vi "Parse Test.vi"() -> ()   [LabVIEW 2015]
uses:
  lib/TOML Value.ctl
  lib/TOML.lvlib
panel:
  out "Parsed Data":T1 {"owner"."dob" format="%<%.3X%z\n%x>T"}
  out "TOML String":string
  in  "Tree":string(tree)
  in  "TOML String":string="# This is a TOML document.\n\ntitle = \"TOML Example\"\n\n[owner]\nname = \"David Taylor\"\ndob = 1991-07-17T07:12:00-07:00 # First class dates\n\n[database]\nserver = \"192.168.1.1\"\nports = [ 8001, 8001, 8002 ]\nconnection_max = 5000\nenabled = true\n\n[servers]\n\n  # Indentation (tabs and/or spaces) is allowed but not required\n  [servers.alpha]\n  ip = \"10.0.0.1\"\n  dc = \"eqdc10\"\n\n  [servers.beta]\n  ip = \"10.0.0.2\"\n  dc = \"eqdc10\"\n\n[clients]\ndata = [ [\"gamma\", \"delta\"], [1, 2] ]\n\n# Line breaks are OK when inside arrays\nhosts = [\n  \"alpha\",\n  \"omega\"\n]\n\n#inline table\ninline_table = {one = 1, two = 2}\n\n[[array_of_tables]]\nmulti-line-string = \"\"\"\nline one\nline two\"\"\"\n\n[[array_of_tables]]\nmulti-line-literal-string = '''\nliteral strings allow special characters \\ unescaped\nline two'''"
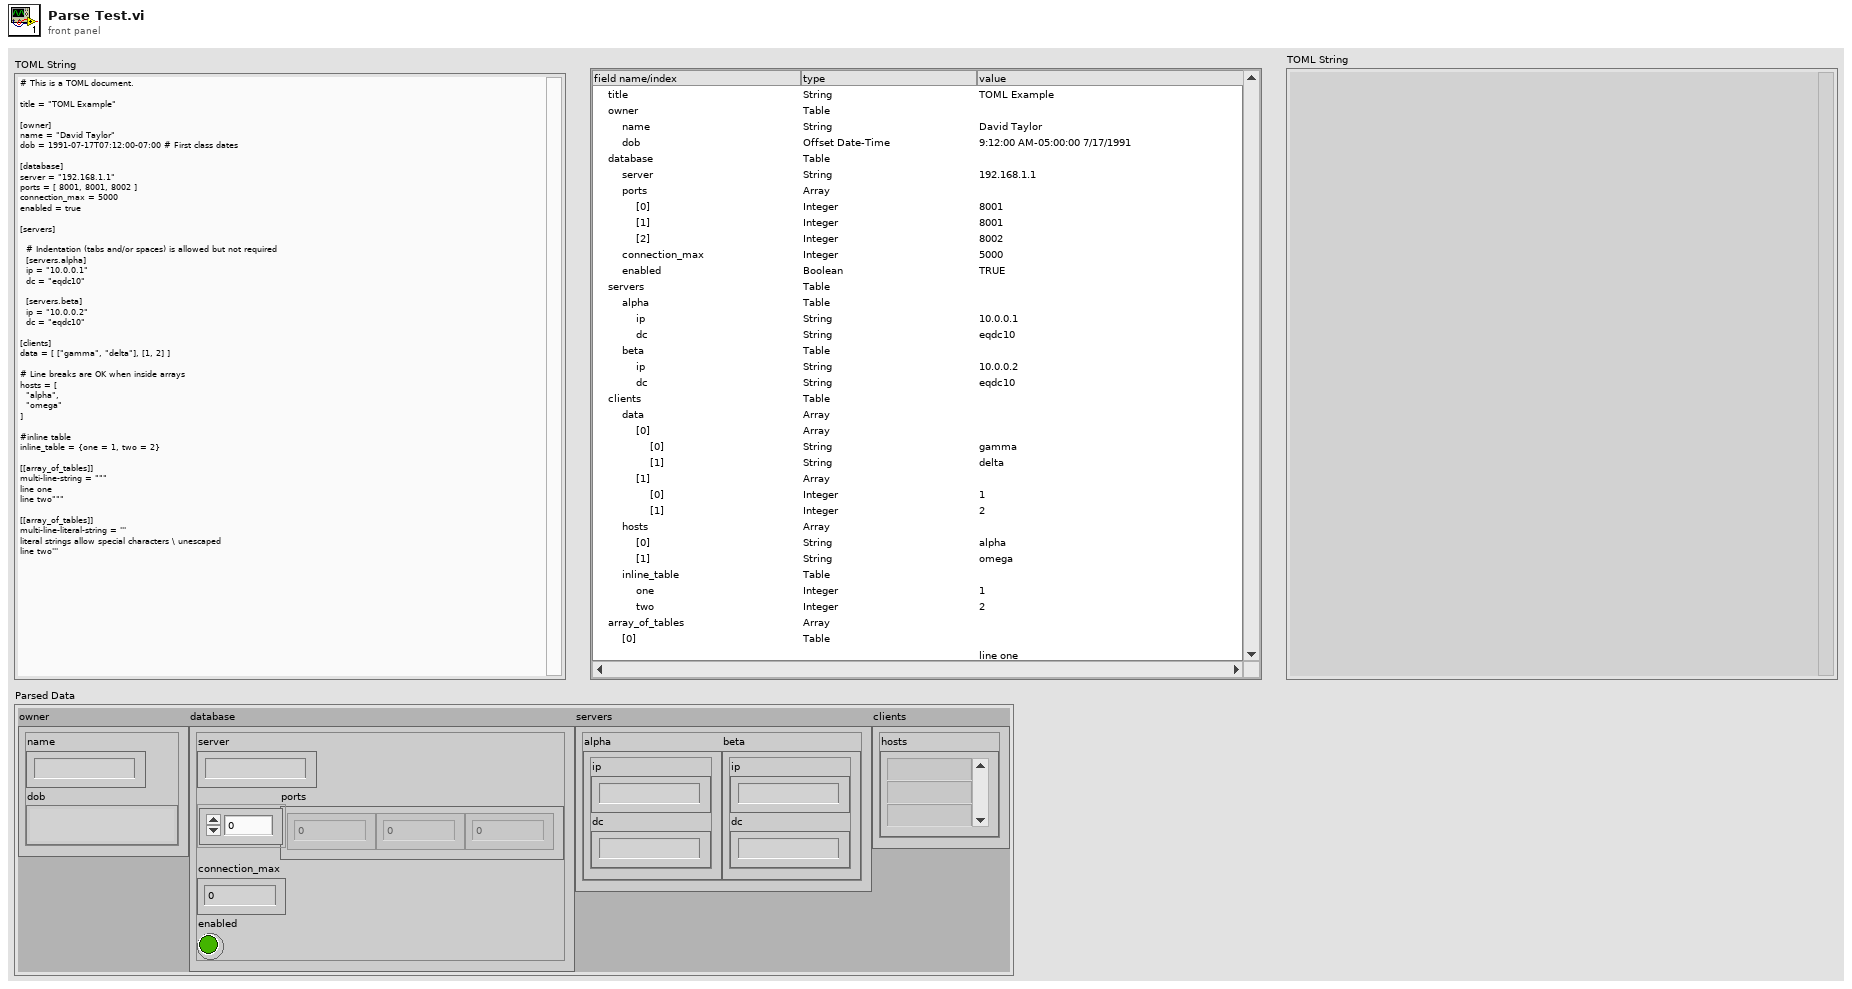
[diagram p1: front panel]
types:
  T1 = cluster{"owner":cluster{"name":string, "dob":timestamp}, "database":cluster{"server":string, "ports":dbl[], "connection_max":dbl, "enabled":bool}, "servers":cluster{"alpha":cluster{"ip":string, "dc":string}, "beta":cluster{"ip":string, "dc":string}}, "clients":cluster{"hosts":string[]}}
  T2 = enum16{"Table", "Array", "String", "Integer", "Float", "Boolean", "Offset Date-Time", "Local Date-Time", "Local Date", "Local Time"}
  T3 = typedef "TOML.lvlib/TOML Value.ctl" = cluster{"\\type":enum16{"Table", "Array", "String", "Integer", "Float", "Boolean", "Offset Date-Time", "Local Date-Time", "Local Date", "Local Time"}, "ÿýÿýÿýÿýÿýÿþÿýÿýÿý\"TOML.lvlib:TOML Key-Value Pair.ctlÿýÿýÿýÿýÿýÿþÿýÿýÿýTOML.lvlib:TOML Value.ctl$$":variant}
  T4 = typedef "TOML.lvlib/TOML Key-Value Pair.ctl" = cluster{"Key":string, "Value":T3}
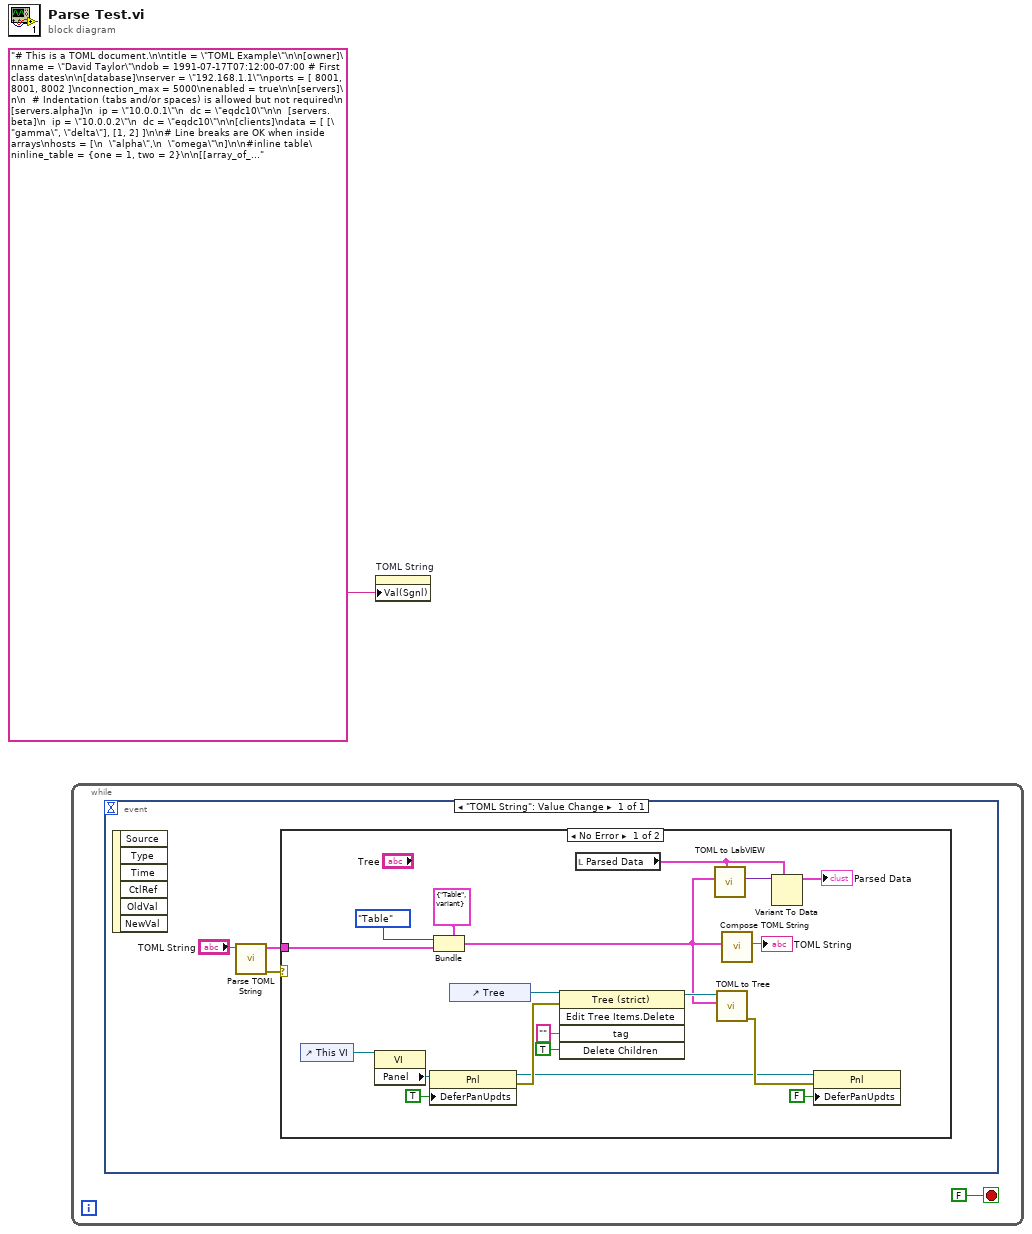
[diagram p0: block diagram]
diagram:
  n1 = while {
    stop <- FALSE stop-if-true
    n2 = event shown="[0] \"TOML String\": Value Change" {
      selector: _ -> [_]
      dyn-events: _ -> [_]
      timeout: _ -> [_]
      event "TOML String": Value Change {
        n3 = event-data() -> ()  [unwired: 1 in, 6 out]
        n4 = call "Parse TOML String.vi"("String"="TOML String") -> ("error out"=w4:errorcluster, "Table"=w5:T4[])  [unwired: 9 in]
        n5 = case shown="No Error" w4 {
          tunnel: w5 -> [w8 _]
          frame No Error {
            n6 = control-ref of="This VI"() -> (w20:refnum<vi>)
            n7 = property class="VI"(reference=w20) -> ("Panel"=w19:refnum<vi>)  [unwired: 1 in, 2 out]
            n8 = property class="Pnl"(reference=w19, "DeferPanUpdts"=TRUE ("Defer Panel Updates")) -> (reference out=w15:refnum<vi>, error out=w17:errorcluster)  [unwired: 1 in]
            n9 = Bundle(cluster=T3 {"\\type"=enum."Table", "ÿýÿýÿýÿýÿýÿþÿýÿýÿý\"TOML.lvlib:TOML Key-Value Pair.ctlÿýÿýÿýÿýÿýÿþÿýÿýÿýTOML.lvlib:TOML Value.ctl$$"=variant} ("Value"), "\\type"=T2."Table" ("Type"), "ÿýÿýÿýÿýÿýÿþÿýÿýÿý\"TOML.lvlib:TOML Key-Value Pair.ctlÿýÿýÿýÿýÿýÿþÿýÿýÿýTOML.lvlib:TOML Value.ctl$$"=w8) -> (w7:T3)
            n10 = control-ref of="Tree"() -> (w24:refnum<vi>)
            n11 = invoke class="Tree (strict)" method="Edit Tree Items.Delete"(reference=w24, error in=w17, "tag"="" ("Tag"), "Delete Children"=TRUE ("Delete Children?")) -> (reference out=w21:refnum<vi>)  [unwired: 1 in, 4 out]
            n12 = local read "Parsed Data"() -> (w12:T1)
            n13 = call "TOML to LabVIEW.vi"("Default Value"=w12, "TOML Value"=w7) -> ("LV Value"=w11:variant)  [unwired: 9 in]
            n14 = call "TOML to Tree.vi"("Value"=w7, "TreeControl in"=w21) -> ("error out"=w16:errorcluster)  [unwired: 9 in]
            n15 = call "Compose TOML String.vi"("Value"=w7) -> ("String"=→"TOML String":string)  [unwired: 10 in]
            n16 = Variant To Data(type=w12, Variant=w11) -> (data=→"Parsed Data":T1)  [unwired: 1 in, 1 out]
            n17 = property class="Pnl"(reference=w15, error in=w16, "DeferPanUpdts"=FALSE ("Defer Panel Updates")) -> ()  [unwired: 2 out]
          }
          frame Error {
          }
        }
      }
    }
  }
  n18 = property on="TOML String" class="Str"("Val(Sgnl)"="# This is a TOML document.\n\ntitle = \"TOML Example\"\n\n[owner]\nname = \"David Taylor\"\ndob = 1991-07-17T07:12:00-07:00 # First class dates\n\n[database]\nserver = \"192.168.1.1\"\nports = [ 8001, 8001, 8002 ]\nconnection_max = 5000\nenabled = true\n\n[servers]\n\n  # Indentation (tabs and/or spaces) is allowed but not required\n  [servers.alpha]\n  ip = \"10.0.0.1\"\n  dc = \"eqdc10\"\n\n  [servers.beta]\n  ip = \"10.0.0.2\"\n  dc = \"eqdc10\"\n\n[clients]\ndata = [ [\"gamma\", \"delta\"], [1, 2] ]\n\n# Line breaks are OK when inside arrays\nhosts = [\n  \"alpha\",\n  \"omega\"\n]\n\n#inline table\ninline_table = {one = 1, two = 2}\n\n[[array_of_tables]]\nmulti-line-string = \"\"\"\nline one\nline two\"\"\"\n\n[[array_of_tables]]\nmulti-line-literal-string = '''\nliteral strings allow special characters \\ unescaped\nline two'''" ("TOML String")) -> ()  [unwired: 2 in, 2 out]
